vi "Write Multiple Coils.vi"(8 "error in (no error)":errorcluster, 9 "coils":bool[](array[boolean]), 10 "starting address":u16, 11 "device data model in":refnum<class "ET-7042UR Data Model.lvclass">) -> (0 "error out":errorcluster, 3 "device data model out":refnum<class "ET-7042UR Data Model.lvclass">)   [LabVIEW 2021, in "ET-7042UR Data Model.lvclass"]
doc: "Writes the values of multiple coils in series, starting at address M."
uses:
  ET-7042UR Data Model.lvclass
  ET-7042UR Data Model.lvclass/ET-7042UR Data Model.ctl
  ICPCON ET Data Model.lvclass
  D:/my_projects/projects/Algorithms/Labview/21/Master CR/Data Model/ICPCON ET7000 Data Model/ICPCON ET Data Model.lvclass
  D:/my_projects/projects/Algorithms/Labview/21/Modbus_v121c/Data Model/Device Data Model.lvclass
  D:/my_projects/projects/Algorithms/Labview/21/Master CR/Data Model/ICPCON ET7000 Data Model/ET-7042UR/ET-7042UR Data Model.lvclass
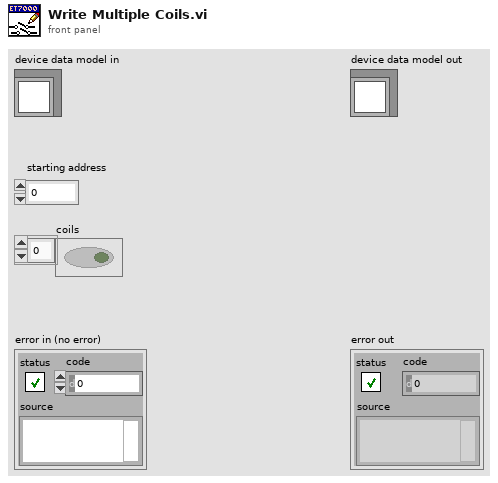
[diagram p1: front panel]
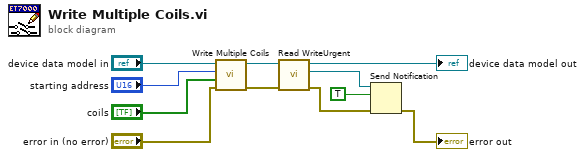
[diagram p0: block diagram]
diagram:
  n1 = call-parent "Write Multiple Coils.vi"("error in (no error)"="error in (no error)", "coils"="coils", "starting address"="starting address", "device data model in"="device data model in") -> ("error out"=w2:errorcluster, "device data model out"=w7:refnum<class "ET-7042UR Data Model.lvclass">)  [unwired: 6 in]
  n2 = call "Read WriteUrgent.vi"("error in (no error)"=w2, "ICPCON ET Data Model in"=w7) -> ("error out"=w4:errorcluster, "WriteUrgent"=w5:refnum<notifier>, "ICPCON ET Data Model out"=→"device data model out":refnum<class "ET-7042UR Data Model.lvclass">)  [unwired: 7 in]
  n3 = Send Notification(notification=TRUE, notifier=w5, error in (no error)=w4) -> (error out=→"error out":errorcluster)  [unwired: 1 out]
